vi "tf FGV.vi"(8 "error in (no error)":errorcluster, 10 "set tf":dbl, 11 "Enum":T1) -> (0 "error out":errorcluster, 3 "tf":dbl)   [LabVIEW 2017, in "admittanceControllerLibrary.lvlib"]
doc: "This FGV contains the final time, which is required for the minimum jerk trajectory."
uses:
  admittanceControllerLibrary.lvlib
  Controls/tf control.ctl
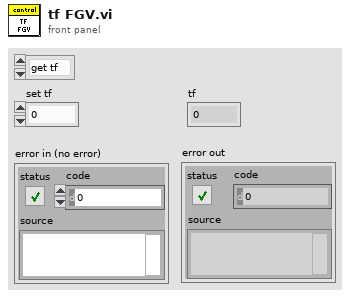
[diagram p1: front panel]
types:
  T1 = typedef "admittanceControllerLibrary.lvlib/tf control.ctl" = enum16{"get tf", "set tf"}
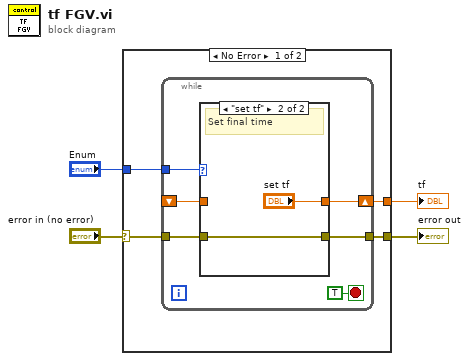
[diagram p0: block diagram]
diagram:
  n1 = case shown="No Error" "error in (no error)" {
    selector: "error in (no error)" -> [w6 w19]
    tunnel: [w8 _] -> w4
    tunnel: "Enum" -> [w7 _]
    tunnel: [w5 w19] -> w1
    frame No Error {
      n2 = while {
        tunnel: w7 -> [w13]
        shift-right: [w12] -> w8
        shift-left: _ -> [w11]
        tunnel: w6 -> [w10]
        tunnel: [w9] -> w5
        stop <- TRUE stop-if-true
        n3 = case shown="\"set tf\"" w13 {
          tunnel: [w16 "set tf"] -> w12
          tunnel: w11 -> [w16 _]
          tunnel: w10 -> [w15 w17]
          tunnel: [w15 w17] -> w9
          frame "get tf", Default {
            # "get final time"
          }
          frame "set tf" {
            # "Set final time"
          }
        }
      }
    }
    frame Error {
    }
  }
  "tf" <- w4
  "error out" <- w1
